vi "pulse Tx.vi"(10 "take it!":bool, 11 "Cluster":T1={"PW"=0, "frequency shift"=0.0, "amp"=0.9999923706054688, "mode type"=0, "mode file"=0, "mode depth"=0, "filter rate_pulse"=0, "filter rate bpsk"=0}) -> (0 "phase":fxp<+/-,16,1>, 1 "frequncy":fxp<+/-,48,0>, 2 "data out":T2, 3 "free dds":bool)   [LabVIEW 2021]
uses:
  <instrlib>/_niInstr/DSP/v1/Shared/Public/IQ Data.ctl
  pdw.ctl
  <instrlib>/_niInstr/Basic Elements/v1/FPGA/Private/Count Up U32.vi
  <instrlib>/_niInstr/DSP/v1/FPGA/Public/Sub VIs/Frequency Shift/Frequency Shift - 1 spc.vi
  <vilib>/rvi/FXPMathLib/FxpAdd/XNode/nifxpmath_Add.xnode
  <instrlib>/_niInstr/DSP/v1/XNodes/Public/Frequency Shift/niInstr DSP v1 Frequency Shift FPGA.xnode
  <instrlib>/_niInstr/DSP/v1/Shared/niInstr DSP v1 Shared.lvlib
  <instrlib>/_niInstr/Basic Elements/v1/FPGA/niInstr Basic Elements v1 FPGA.lvlib
  <vilib>/rvi/FXPMathLib/sim/FxpSim.dll
  <instrlib>/_niInstr/DSP/v1/FPGA/niInstr DSP v1 FPGA.lvlib
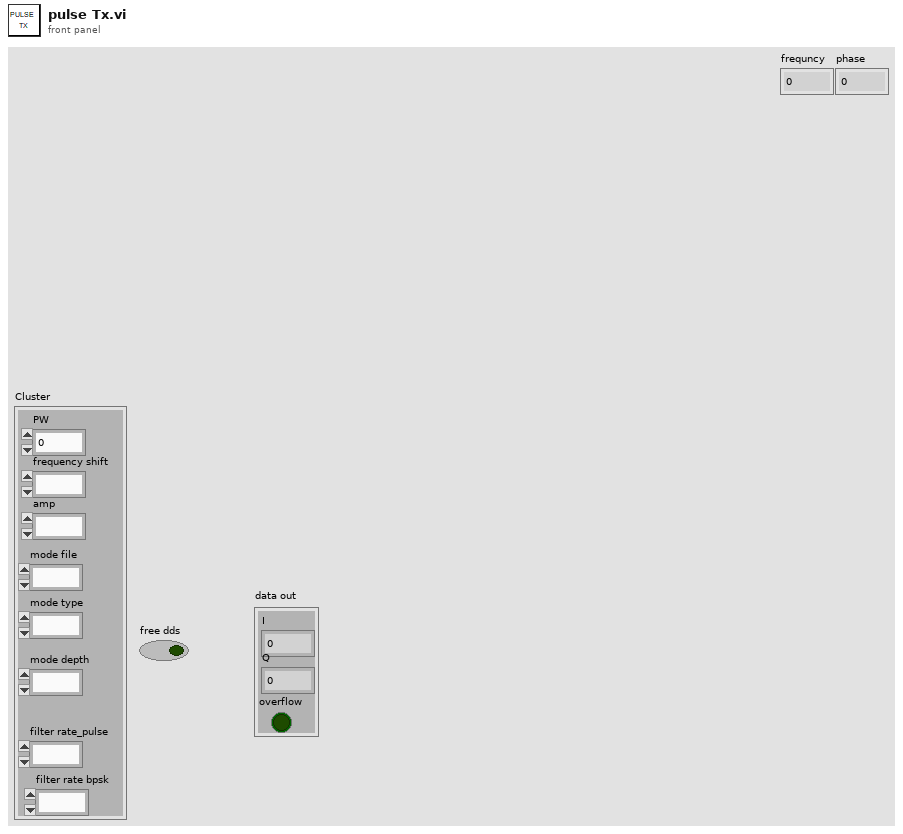
[diagram p1: front panel]
types:
  T1 = typedef "pdw.ctl" = cluster{"PW":u32, "frequency shift":fxp<+/-,48,0>, "amp":fxp<+/-,18,1>, "mode type":u8, "mode file":u8, "mode depth":u32, "filter rate_pulse":u16, "filter rate bpsk":u16}
  T2 = typedef "niInstr DSP v1 Shared.lvlib/IQ Data.ctl" = cluster{"I":fxp<+/-,18,1>, "Q":fxp<+/-,18,1>, "overflow":bool}
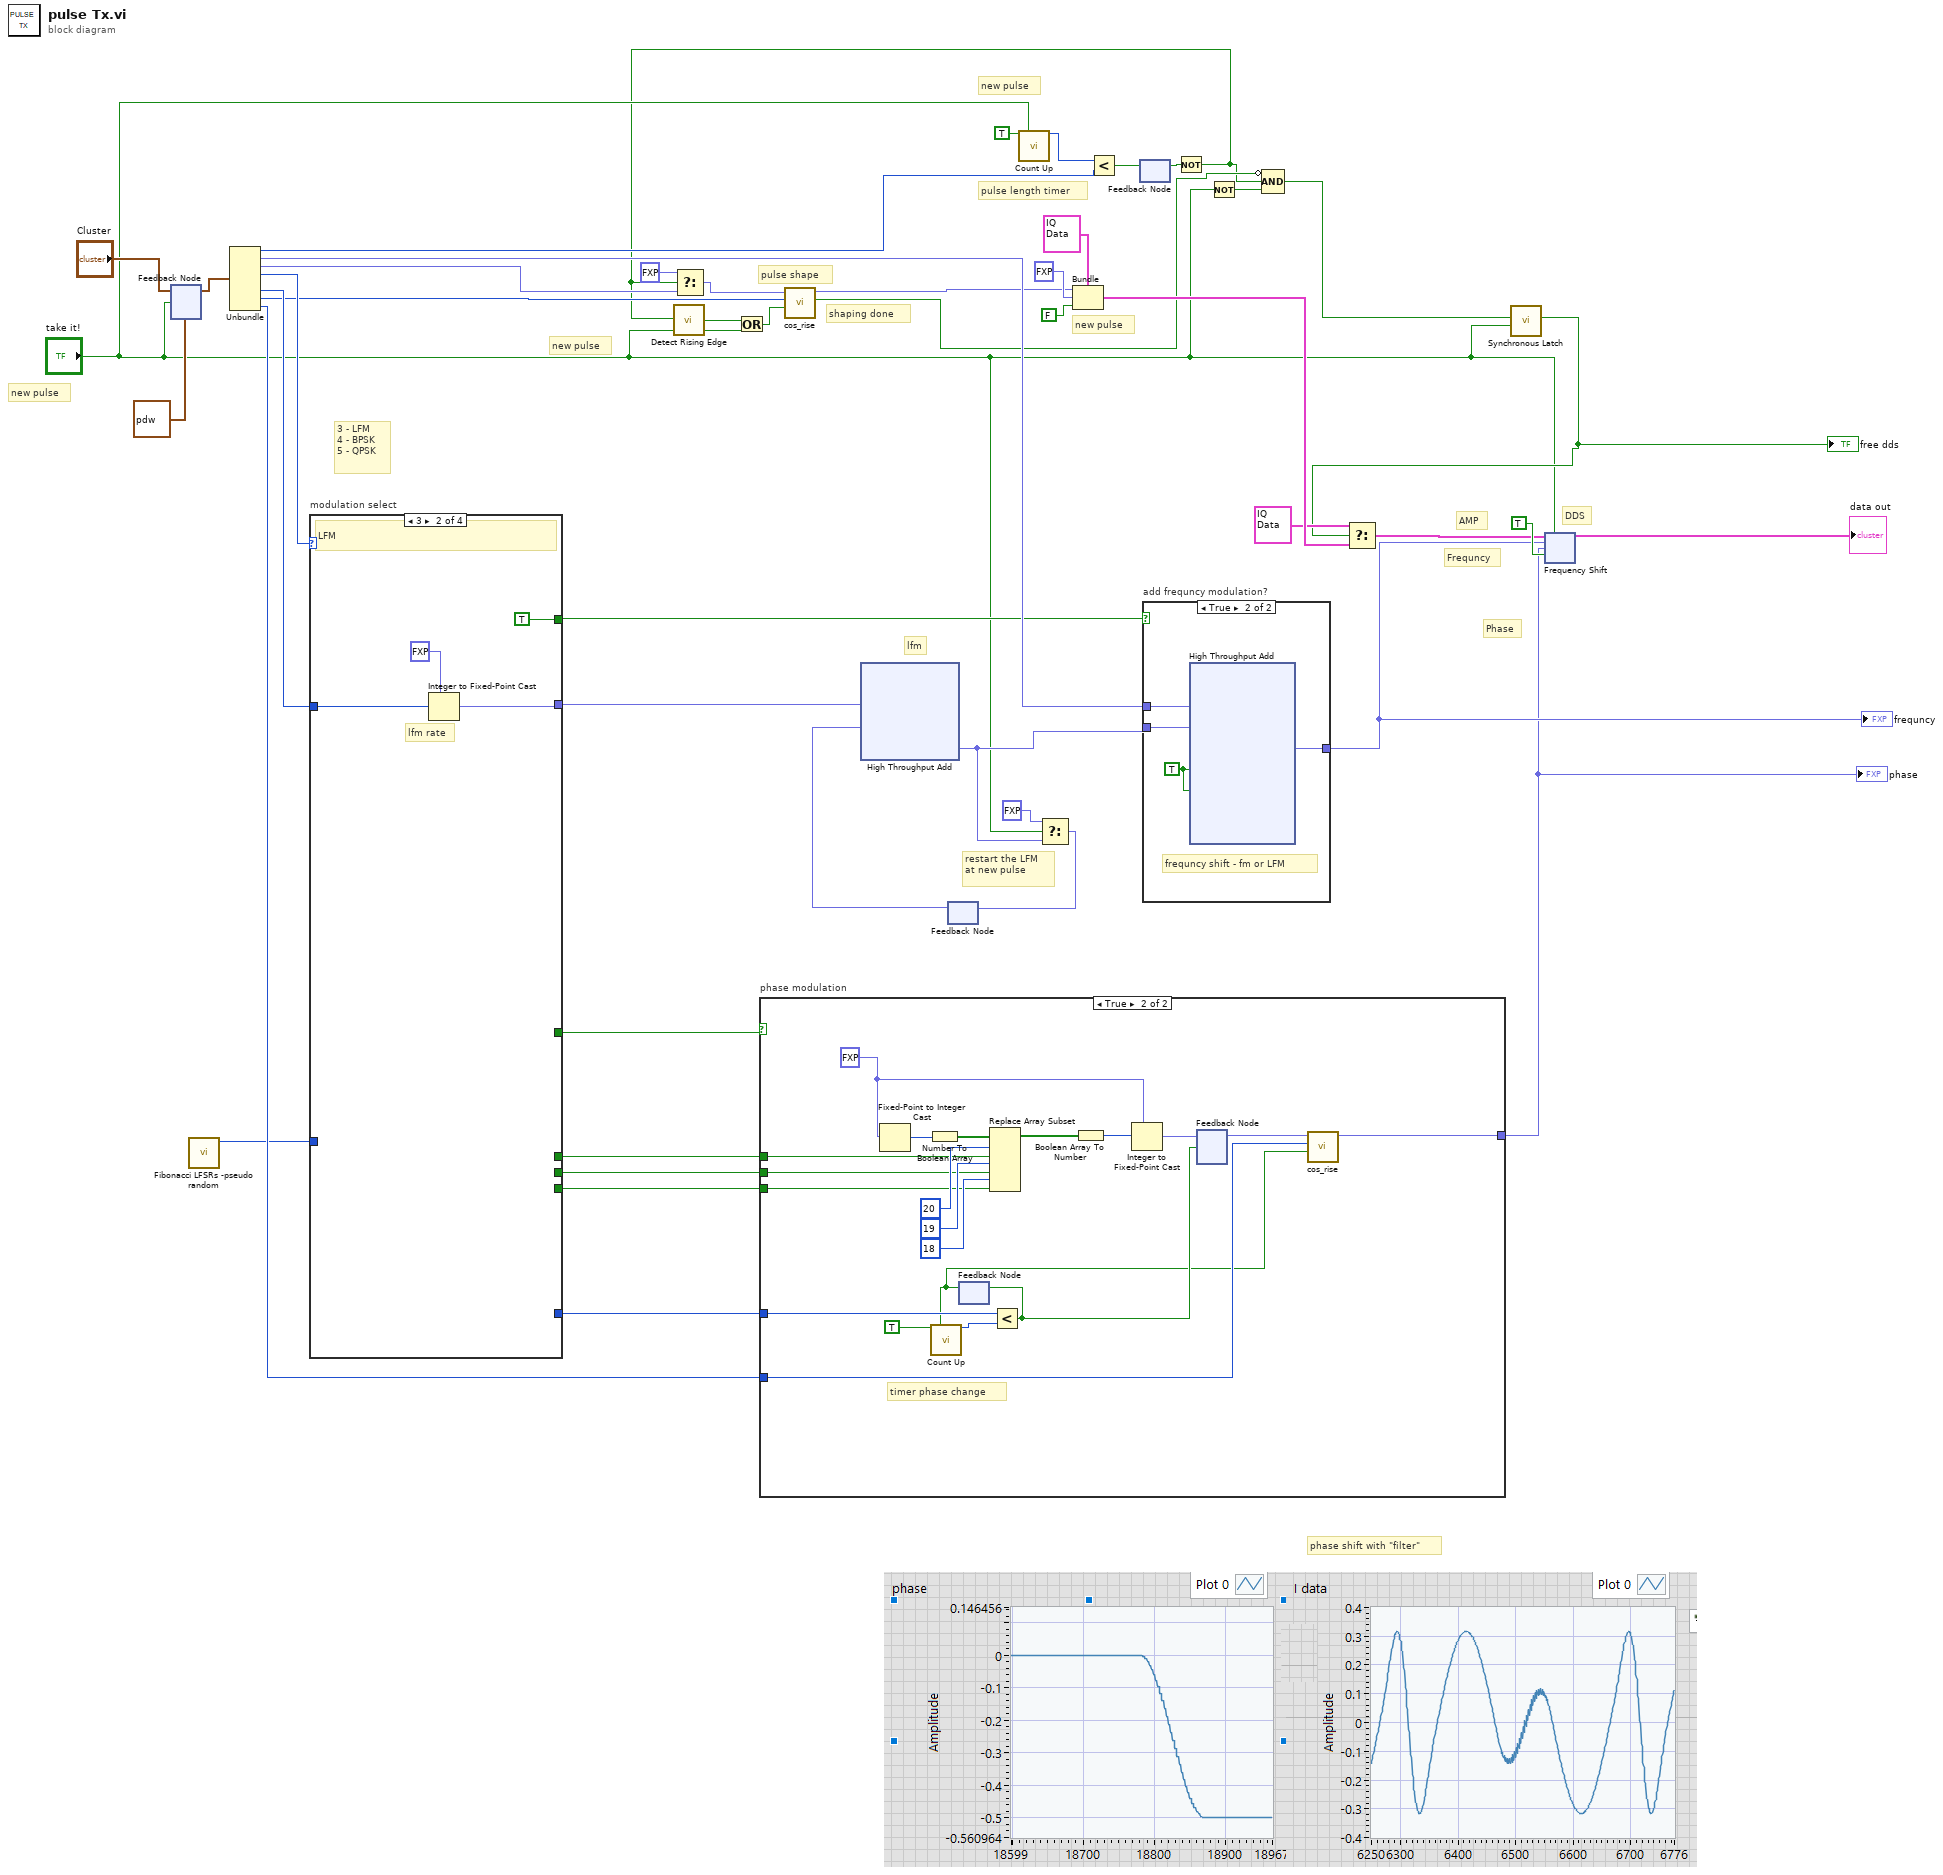
[diagram p0: block diagram]
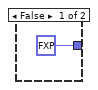
[diagram p2: hidden frame]
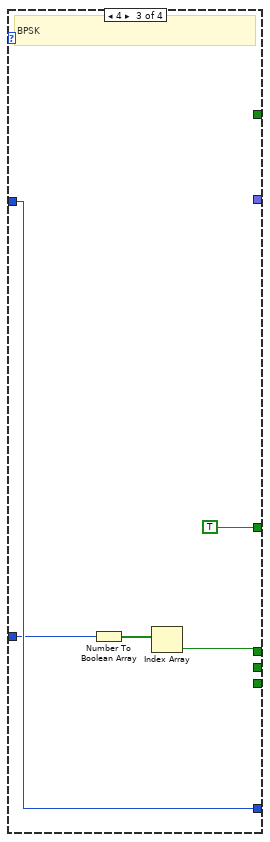
[diagram p5: hidden frame]
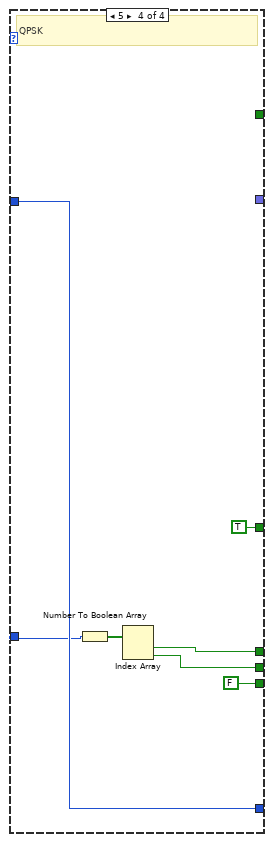
[diagram p6: hidden frame]
diagram:
  # "phase shift with \"filter\""
  # "Phase"
  # "Frequncy"
  # "AMP"
  # "DDS"
  # "shaping done"
  # "3 - LFM\n4 - BPSK\n5 - QPSK"
  # "pulse length timer"
  # "restart the LFM\nat new pulse"
  # "lfm"
  # "pulse shape"
  # "new pulse"
  # "new pulse"
  # "new pulse"
  # "new pulse"
  n1 = feedback #1(T1 {"PW"=0, "frequency shift"=0.0, "amp"=0.9999923706054688, "mode type"=0, "mode file"=0, "mode depth"=0, "filter rate_pulse"=0, "filter rate bpsk"=0} ("Cluster")) -> (w40:T1)
  n2 = feedback-in #1("Cluster", "take it!") -> ()
  n3 = call "Fibonacci LFSRs -pseudo random.vi"() -> ("rand number"=w6:u16)  [unwired: 11 in]
  n4 = Unbundle(w40) -> ("PW"=w45:u32, "frequency shift"=w35:fxp<+/-,48,0>, "amp"=w9:fxp<+/-,18,1>, "mode type"=w37:u8, "mode depth"=w36:u32, "filter rate_pulse"=w11:u16, "filter rate bpsk"=w17:u16)  [unwired: 1 out]
  n5 = case "modulation select" shown="3" w37 {
    tunnel: w36 -> [_ w50 w53 w58]
    tunnel: [_ w49 _ _] -> w30
    tunnel: [_ TRUE ("s") _ _] -> w27
    tunnel: [_ _ _ FALSE] -> w25
    tunnel: [_ _ _ w60] -> w24
    tunnel: [_ _ w55 w62] -> w23
    tunnel: [_ _ TRUE TRUE] -> w22
    tunnel: [_ _ w53 w58] -> w21
    tunnel: w6 -> [_ _ w52 w57]
    frame Default {
    }
    frame 3 {
      # "lfm rate"
      # "LFM"
      n6 = Integer to Fixed-Point Cast(fixed-point type=fxp<+,32,-16> 0.0, integer=w50) -> (fixed-point=w49:fxp<+,32,-16>)
    }
    frame 4 {
      # "BPSK"
      n7 = Number To Boolean Array(number=w52) -> (Boolean array=w56:bool[])
      n8 = Index Array(array=w56) -> (element=w55:bool)  [unwired: 1 in]
    }
    frame 5 {
      # "QPSK"
      n9 = Number To Boolean Array(number=w57) -> (Boolean array=w63:bool[])
      n10 = Index Array(array=w63) -> (element #1=w62:bool, element #2=w60:bool)  [unwired: 2 in]
    }
  }
  n11 = case "phase modulation" shown="True" w22 {
    tunnel: w25 -> [_ w76]
    tunnel: w24 -> [_ w75]
    tunnel: w23 -> [_ w74]
    tunnel: w21 -> [_ w72]
    tunnel: [fxp<+/-,16,1> 0.0 ("filter out") w67] -> w18
    tunnel: w17 -> [_ w66]
    frame False {
    }
    frame True {
      w78 = fxp<+/-,21,0> 0.0 ("phase")
      # "timer phase change"
      n12 = Fixed-Point to Integer Cast(1:w78) -> (0:w84:i32)
      n13 = Number To Boolean Array(number=w84) -> (Boolean array=w82:bool[])
      n14 = feedback #2() -> (w65:bool)  [unwired: 1 in]
      n15 = call-poly <instrlib>:"Count Up.vi"("increment"=TRUE, "reset"=w65) -> ("count out"=w71:u32)  [unwired: 13 in]
      n16 = Replace Array Subset(array=w82, new element #1=w74, index #1=20 ("index"), new element #2=w75, index #2=19 ("index"), new element #3=w76, index #3=18 ("index")) -> (w77:bool[])
      n17 = Less?(x=w72, y=w71) -> (x < y?=w69:bool)
      n18 = feedback-in #2(w69) -> ()
      n19 = Boolean Array To Number(Boolean array=w77) -> (number=w83:u32)
      n20 = Integer to Fixed-Point Cast(fixed-point type=w78, integer=w83) -> (fixed-point=w73:fxp<+/-,21,0>)
      n21 = feedback-in #3(w73, w69) -> ()
      n22 = feedback #3() -> (w68:fxp<+/-,21,0>)  [unwired: 1 in]
      n23 = call "cos_rise.vi"("new step"=w65, "change rate"=w66, "data in"=w68) -> ("data out"=w67:fxp<+/-,16,1>)  [unwired: 7 in, 1 out]
    }
  }
  "phase" <- w18
  n24 = feedback #4() -> (w29:fxp<+/-,48,0>)  [unwired: 1 in]
  n25 = xnode ("High Throughput Add")("x"=w30, "y"=w29) -> ("x+y"=w28:fxp<+/-,48,0>)
  n26 = call-poly <instrlib>:"Count Up.vi"("increment"=TRUE, "reset"="take it!") -> ("count out"=w20:u32)  [unwired: 13 in]
  n27 = Select(t=fxp<+/-,48,0> 0.0, s="take it!", f=w28) -> (s? t:f=w31:fxp<+/-,48,0>)
  n28 = feedback-in #4(w31) -> ()
  n29 = Less?(x=w20, y=w45) -> (x < y?=w19:bool)
  n30 = feedback #5() -> (w16:bool)  [unwired: 1 in]
  n31 = feedback-in #5(w19) -> ()
  n32 = case "add frequncy modulation?" shown="True" w27 {
    tunnel: w35 -> [w85 w89]
    tunnel: w28 -> [_ w88]
    tunnel: [w85 w87] -> w32
    frame False {
    }
    frame True {
      w86 = TRUE ("input valid")
      # "frequncy shift - fm or LFM"
      n33 = xnode ("High Throughput Add")("x"=w89, "y"=w88, "input valid"=w86, "ready for output (T)"=w86) -> ("x+y"=w87:fxp<+/-,48,0>)  [unwired: 2 out]
    }
  }
  "frequncy" <- w32
  n34 = Not(x=w16) -> (.not. x?=w2:bool)
  n35 = call <instrlib>:"Detect Rising Edge.vi"("signal"=w2) -> ("edge detected"=w1:bool)  [unwired: 14 in]
  n36 = Select(t=fxp<+/-,18,1> 0.0, s=w2, f=w9) -> (s? t:f=w8:fxp<+/-,18,1>)
  n37 = Or(x=w1, y="take it!") -> (x .or. y?=w3:bool)
  n38 = call "cos_rise.vi"("new step"=w3, "change rate"=w11, "data in"=w8) -> ("steping"=w10:bool, "data out"=w5:fxp<+/-,16,1>)  [unwired: 7 in]
  n39 = Bundle(cluster=T2 {"I"=0.9999923706054688, "Q"=0.0, "overflow"=FALSE} ("data"), "I"=w5, "Q"=fxp<+/-,18,1> 0.0, "overflow"=FALSE ("input valid")) -> (w15:T2)
  n40 = Not(x="take it!") -> (.not. x?=w39:bool)
  n41 = Compound Arithmetic op=AND(invert w10, w2, w39) -> (w38:bool)
  n42 = call <instrlib>:"Synchronous Latch.vi"("clear"="take it!", "set"=w38) -> ("out"=w13:bool)  [unwired: 9 in]
  "free dds" <- w13
  n43 = Select(t=T2 {"I"=0.0, "Q"=0.0, "overflow"=FALSE}, s=w13, f=w15) -> (s? t:f=w12:T2)
  n44 = xnode "Frequency Shift"("data in"=w12, "reset"="take it!", "frequency shift"=w32, "phase"=w18, "input valid"=TRUE) -> ("data out"=→"data out":T2)  [unwired: 1 in, 2 out]
